vi "Queued State Machine with UI Event Handling.vi"() -> ()   [LabVIEW 2010]
doc: "이 VI는 큐 기반 상태 머신의 템플릿입니다. 프로세스 1 및 프로세스 2를 사용자의 상태로 대체하십시오. 더 많은 프로세스를 추가하려면, 타입 정의된 열거형 상수를 수정하십시오. 열거형 순서는 클러스터 순서와 일치해야 합니다."
uses:
  State Enum.ctl
panel:
  in  "정지":bool
  in  "프로세스 2":bool
  in  "프로세스 1":bool
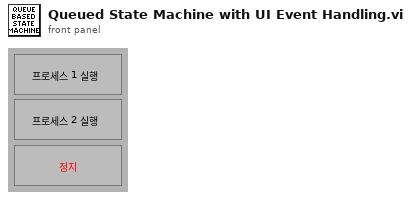
[diagram p1: front panel]
types:
  T1 = typedef "State Enum.ctl" = enum32{"이벤트 기다림", "프로세스 1", "프로세스 2", "정지"}
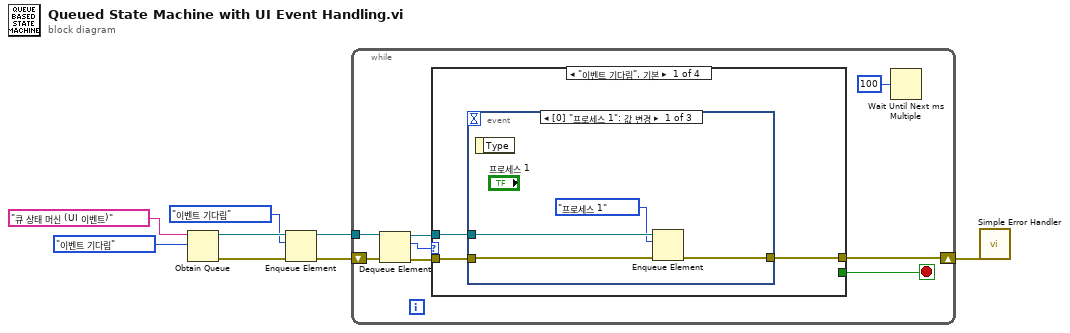
[diagram p0: block diagram]
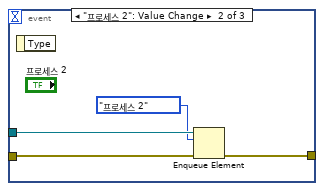
[diagram p2: hidden frame]
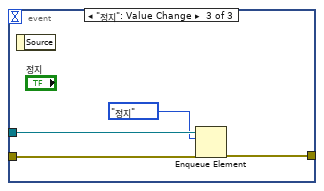
[diagram p3: hidden frame]
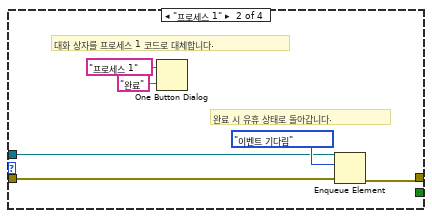
[diagram p4: hidden frame]
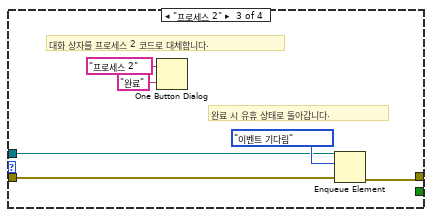
[diagram p5: hidden frame]
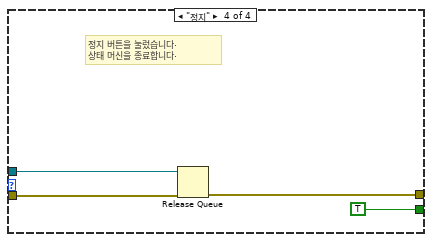
[diagram p6: hidden frame]
diagram:
  n1 = Obtain Queue(name (unnamed)="큐 상태 머신 (UI 이벤트)", element data type=State_Enum."이벤트 기다림" ("Enum")) -> (queue out=w6:refnum<queue>, error out=w7:errorcluster)  [unwired: 3 in, 1 out]
  n2 = Enqueue Element(queue=w6, element=State_Enum."이벤트 기다림" ("Enum"), error in (no error)=w7) -> (queue out=w4:refnum<queue>, error out=w5:errorcluster)  [unwired: 2 out]
  n3 = while {
    tunnel: w4 -> [w11]
    shift-right: [w14] -> w1
    shift-left: w5 -> [w13]
    stop <- w16 stop-if-true
    n4 = Dequeue Element(queue=w11, error in (no error)=w13) -> (queue out=w10:refnum<queue>, element=w9:T1, error out=w12:errorcluster)  [unwired: 2 out]
    n5 = case shown="\"이벤트 기다림\", 기본" w9 {
      tunnel: [_ _ _ TRUE] -> w16
      tunnel: w12 -> [w18 w35 w41 w46]
      tunnel: w10 -> [w19 w32 w38 w45]
      tunnel: [w17 w34 w40 w44] -> w14
      frame "이벤트 기다림", Default {
        n6 = event shown="[0] \"프로세스 1\": 값 변경" {
          selector: _ -> [_ _ _]
          dyn-events: _ -> [_ _ _]
          timeout: _ -> [_ _ _]
          tunnel: w19 -> [w23 w27 w31]
          tunnel: w18 -> [w22 w26 w30]
          tunnel: [w21 w25 w29] -> w17
          event "프로세스 1": Value Change {
            n7 = event-data() -> ()  [unwired: 2 out]
            n8 = Enqueue Element(queue=w23, element=State_Enum."프로세스 1" ("Enum"), error in (no error)=w22) -> (error out=w21:errorcluster)  [unwired: 1 in, 2 out]
          }
          event "프로세스 2": Value Change {
            n9 = event-data() -> ()  [unwired: 2 out]
            n10 = Enqueue Element(queue=w27, element=State_Enum."프로세스 2" ("Enum"), error in (no error)=w26) -> (error out=w25:errorcluster)  [unwired: 1 in, 2 out]
          }
          event "정지": Value Change {
            n11 = event-data() -> ()  [unwired: 2 out]
            n12 = Enqueue Element(queue=w31, element=State_Enum."정지" ("Enum"), error in (no error)=w30) -> (error out=w29:errorcluster)  [unwired: 1 in, 2 out]
          }
        }
      }
      frame "프로세스 1" {
        # "완료 시 유휴 상태로 돌아갑니다."
        # "대화 상자를 프로세스 1 코드로 대체합니다."
        n13 = One Button Dialog(message="프로세스 1", button name ("OK")="완료") -> ()  [unwired: 1 out]
        n14 = Enqueue Element(queue=w32, element=State_Enum."이벤트 기다림" ("Enum"), error in (no error)=w35) -> (error out=w34:errorcluster)  [unwired: 3 out]
      }
      frame "프로세스 2" {
        # "완료 시 유휴 상태로 돌아갑니다."
        # "대화 상자를 프로세스 2 코드로 대체합니다."
        n15 = One Button Dialog(message="프로세스 2", button name ("OK")="완료") -> ()  [unwired: 1 out]
        n16 = Enqueue Element(queue=w38, element=State_Enum."이벤트 기다림" ("Enum"), error in (no error)=w41) -> (error out=w40:errorcluster)  [unwired: 3 out]
      }
      frame "정지" {
        # "정지 버튼을 눌렀습니다.\n상태 머신을 종료합니다."
        n17 = Release Queue(queue=w45, error in (no error)=w46) -> (error out=w44:errorcluster)  [unwired: 1 in, 2 out]
      }
    }
    n18 = Wait Until Next ms Multiple(millisecond multiple=u32 100) -> ()  [unwired: 1 out]
  }
  n19 = call <vilib>:"Simple Error Handler.vi"("error in (no error)"=w1) -> ()  [unwired: 1 in, 8 out]
